vi "Files_names.vi"(2 "actualSamples\narray":i32[](array[numeric]), 3 "Type of\nmeasurement":T1, 4 "Name root":string, 5 "File location":path) -> (0 "Files path array":path[](array[path]), 1 "Files name array":string[](array[string]))   [LabVIEW 2013]
uses:
  Strict Type Defs/type_meas_enum.ctl
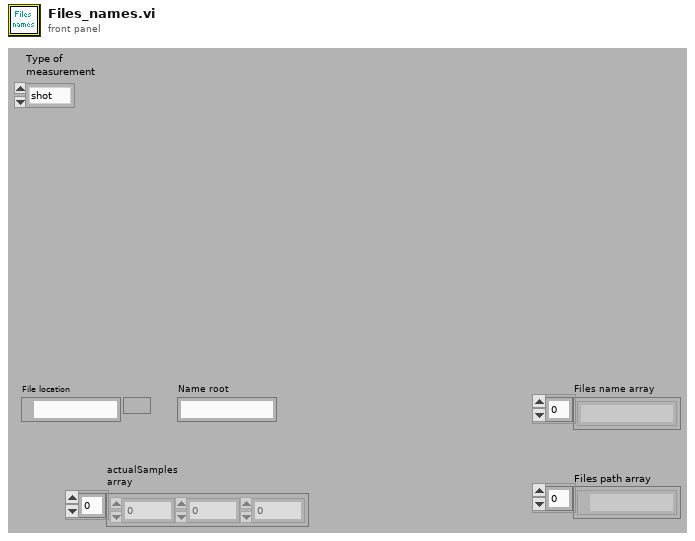
[diagram p1: front panel]
types:
  T1 = typedef "type_meas_enum.ctl" = enum16{"shot", "x", "p", "electronic"}
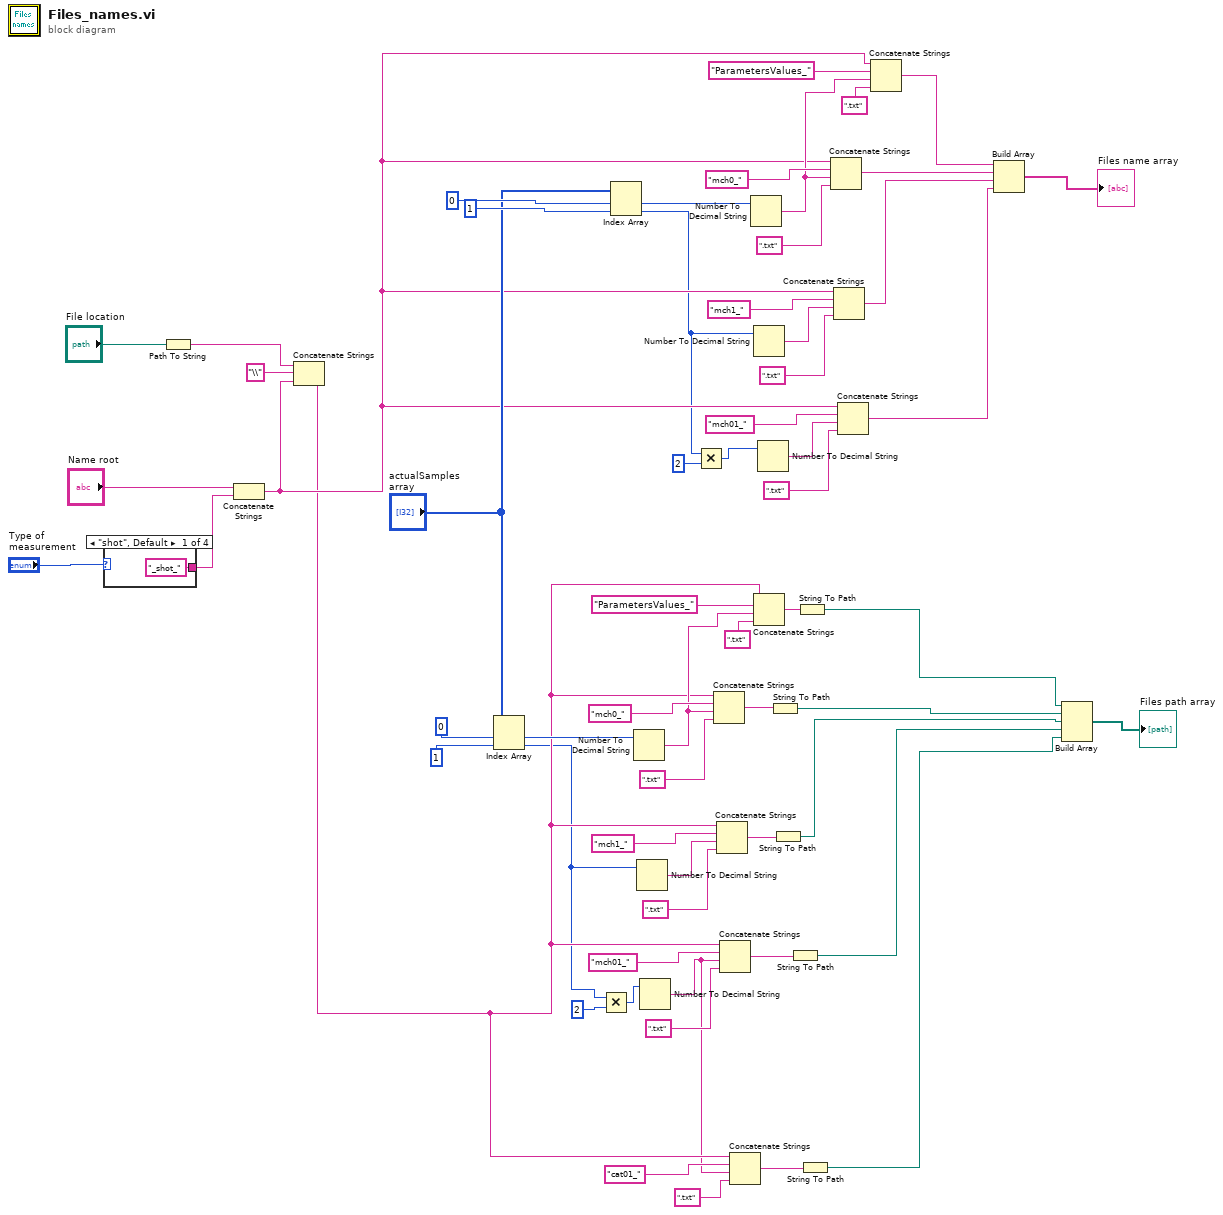
[diagram p0: block diagram]
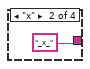
[diagram p2: hidden frame]
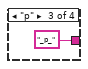
[diagram p3: hidden frame]
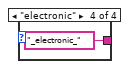
[diagram p4: hidden frame]
diagram:
  n1 = case shown="\"shot\", Default" "Type of\nmeasurement" {
    tunnel: ["_shot_" "_x_" "_p_" "_electronic_"] -> w46
    frame "shot", Default {
    }
    frame "x" {
    }
    frame "p" {
    }
    frame "electronic" {
    }
  }
  n2 = Path To String(path="File location") -> (string=w31:string)
  n3 = Concatenate Strings("Name root", w46) -> (w14:string)
  n4 = Concatenate Strings(w31, "\\" ("string"), w14) -> (w6:string)
  n5 = Index Array(array="actualSamples\narray", index #1=0 ("index"), index #2=1 ("index")) -> (element #1=w53:i32, element #2=w5:i32)
  n6 = Multiply(x=w5, y=2) -> (x*y=w4:i32)
  n7 = Index Array(array="actualSamples\narray", index #1=0 ("index"), index #2=1 ("index")) -> (element #1=w38:i32, element #2=w13:i32)
  n8 = Number To Decimal String(number=w53) -> (decimal integer string=w45:string)  [unwired: 1 out]
  n9 = Number To Decimal String(number=w5) -> (decimal integer string=w51:string)  [unwired: 1 out]
  n10 = Number To Decimal String(number=w4) -> (decimal integer string=w3:string)  [unwired: 1 out]
  n11 = Multiply(x=w13, y=2) -> (x*y=w12:i32)
  n12 = Concatenate Strings(w6, "mch0_" ("string"), w45, ".txt") -> (w49:string)
  n13 = Concatenate Strings(w6, "mch1_" ("string"), w51, ".txt") -> (w48:string)
  n14 = Concatenate Strings(w6, "mch01_" ("string"), w3, ".txt") -> (w20:string)
  n15 = Concatenate Strings(w6, "cat01_" ("string"), w3, ".txt") -> (w7:string)
  n16 = Number To Decimal String(number=w38) -> (decimal integer string=w34:string)  [unwired: 1 out]
  n17 = Number To Decimal String(number=w13) -> (decimal integer string=w36:string)  [unwired: 1 out]
  n18 = Concatenate Strings(w6, "ParametersValues_" ("string"), w45, ".txt" ("string")) -> (w60:string)
  n19 = Number To Decimal String(number=w12) -> (decimal integer string=w17:string)  [unwired: 1 out]
  n20 = String To Path(string=w49) -> (path=w25:path)
  n21 = String To Path(string=w48) -> (path=w26:path)
  n22 = String To Path(string=w20) -> (path=w19:path)
  n23 = String To Path(string=w60) -> (path=w24:path)
  n24 = String To Path(string=w7) -> (path=w2:path)
  n25 = Concatenate Strings(w14, "mch0_" ("string"), w34, ".txt") -> (w30:string)
  n26 = Concatenate Strings(w14, "mch1_" ("string"), w36, ".txt") -> (w28:string)
  n27 = Concatenate Strings(w14, "mch01_" ("string"), w17, ".txt") -> (w15:string)
  n28 = Concatenate Strings(w14, "ParametersValues_" ("string"), w34, ".txt" ("string")) -> (w29:string)
  n29 = Build Array(w29, w30, w28, w15) -> (→"Files name array":string[])
  n30 = Build Array(w24, w25, w26, w19, w2) -> (→"Files path array":path[])
